vi "Check condizioni gestione tabelle.vi"(10 "Array 2":T1(array[cluster]) {"Medie RT" min=-1 max=100; "decimali" min=-1 max=5}) -> (3 "condizioni ok":bool)   [LabVIEW 2019]
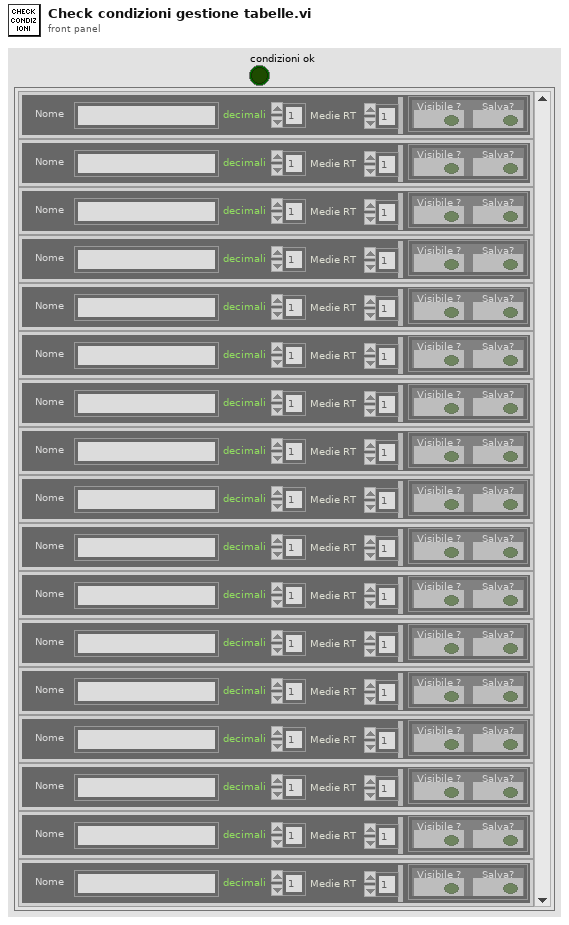
[diagram p1: front panel]
types:
  T1 = cluster{"Nome":string, "QH":cluster{"Visibile ?":bool, "Salva?":bool}, "decimali":i8, "Medie RT":i8}[]
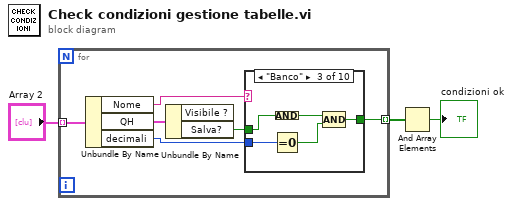
[diagram p0: block diagram]
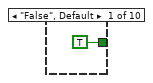
[diagram p2: hidden frame]
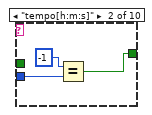
[diagram p3: hidden frame]
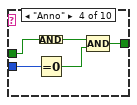
[diagram p4: hidden frame]
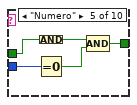
[diagram p5: hidden frame]
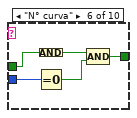
[diagram p6: hidden frame]
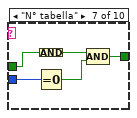
[diagram p7: hidden frame]
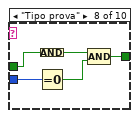
[diagram p8: hidden frame]
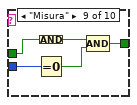
[diagram p9: hidden frame]
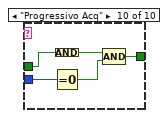
[diagram p10: hidden frame]
diagram:
  n1 = for {
    tunnel: "Array 2" -> [w9] mode=indexing
    tunnel: [w4] -> w3 mode=indexing
    n2 = Unbundle By Name(w9) -> ("Nome"=w7:string, "QH"=w8:cluster{"Visibile ?":bool, "Salva?":bool}, "decimali"=w6:i8)
    n3 = Unbundle By Name(w8) -> ("Salva?"=w5:bool)  [unwired: 1 out]
    n4 = case shown="\"Banco\"" w7 {
      tunnel: w6 -> [_ w13 w18 w23 w28 w33 w38 w43 w48 w53]
      tunnel: w5 -> [_ _ w17 w22 w27 w32 w37 w42 w47 w52]
      tunnel: [TRUE w11 w14 w19 w24 w29 w34 w39 w44 w49] -> w4
      frame "False", Default {
      }
      frame "tempo[h:m:s]" {
        n5 = Equal?(x=i8 -1, y=w13) -> (x = y?=w11:bool)
      }
      frame "Banco" {
        n6 = Equal To 0?(x=w18) -> (x = 0?=w16:bool)
        n7 = Compound Arithmetic op=AND(w17) -> (w15:bool)
        n8 = Compound Arithmetic op=AND(w15, w16) -> (w14:bool)
      }
      frame "Anno" {
        n9 = Equal To 0?(x=w23) -> (x = 0?=w21:bool)
        n10 = Compound Arithmetic op=AND(w22) -> (w20:bool)
        n11 = Compound Arithmetic op=AND(w20, w21) -> (w19:bool)
      }
      frame "Numero" {
        n12 = Equal To 0?(x=w28) -> (x = 0?=w26:bool)
        n13 = Compound Arithmetic op=AND(w27) -> (w25:bool)
        n14 = Compound Arithmetic op=AND(w25, w26) -> (w24:bool)
      }
      frame "N° curva" {
        n15 = Equal To 0?(x=w33) -> (x = 0?=w31:bool)
        n16 = Compound Arithmetic op=AND(w32) -> (w30:bool)
        n17 = Compound Arithmetic op=AND(w30, w31) -> (w29:bool)
      }
      frame "N° tabella" {
        n18 = Equal To 0?(x=w38) -> (x = 0?=w36:bool)
        n19 = Compound Arithmetic op=AND(w37) -> (w35:bool)
        n20 = Compound Arithmetic op=AND(w35, w36) -> (w34:bool)
      }
      frame "Tipo prova" {
        n21 = Equal To 0?(x=w43) -> (x = 0?=w41:bool)
        n22 = Compound Arithmetic op=AND(w42) -> (w40:bool)
        n23 = Compound Arithmetic op=AND(w40, w41) -> (w39:bool)
      }
      frame "Misura" {
        n24 = Equal To 0?(x=w48) -> (x = 0?=w46:bool)
        n25 = Compound Arithmetic op=AND(w47) -> (w45:bool)
        n26 = Compound Arithmetic op=AND(w45, w46) -> (w44:bool)
      }
      frame "Progressivo Acq" {
        n27 = Equal To 0?(x=w53) -> (x = 0?=w51:bool)
        n28 = Compound Arithmetic op=AND(w52) -> (w50:bool)
        n29 = Compound Arithmetic op=AND(w50, w51) -> (w49:bool)
      }
    }
  }
  n30 = And Array Elements(Boolean array=w3) -> (logical AND=→"condizioni ok":bool)
